vi "Do.vi"(8 "error in (no error)":errorcluster, 10 "Actor in":refnum<class "Actor.lvclass">, 11 "Initiate Sample Transfer Msg":refnum<class "Initiate Sample Transfer Msg.lvclass">) -> (0 "error out":errorcluster, 2 "Actor out":refnum<class "Actor.lvclass">)   [LabVIEW 2015, in "cRIO-Carbondioxide.lvlib" / "cRIO-CO2.lvlib" / "Initiate Sample Transfer Msg.lvclass"]
doc: "This VI delivers the message to the actor by calling the appropriate method(s) on the actor."
uses:
  Initiate Sample Transfer Msg.lvclass
  <vilib>/ActorFramework/Actor/Actor.lvclass
  cRIO-CO2/cRIO-CO2.lvclass
  Initiate Sample Transfer Msg.lvclass/Initiate Sample Transfer Msg.ctl
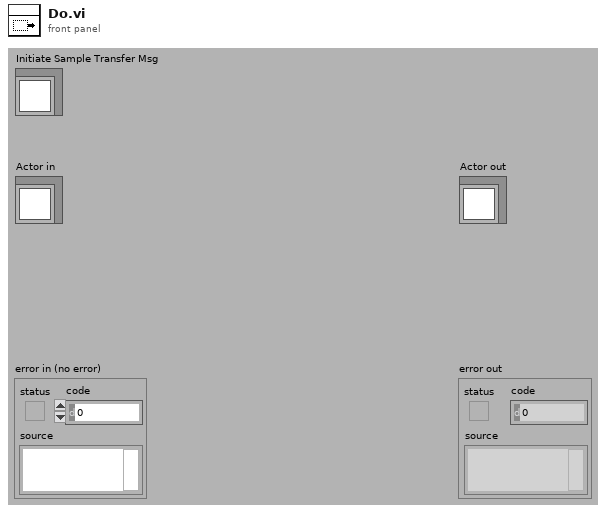
[diagram p1: front panel]
types:
  T1 = typedef "Sample Transfer Container Enumerator.ctl" = enum16{"None", "Sample 1", "Sample 2", "Sample 3", "Sample 4", "Sample 5", "Storage 01", "Storage 02", "Storage 03", "Storage 04", "Storage 05", "Storage 06", "Storage 07", "Storage 08", "Storage 09", "Storage 10", "Storage 11", "Storage 12", "Syringe", "Undefined"}
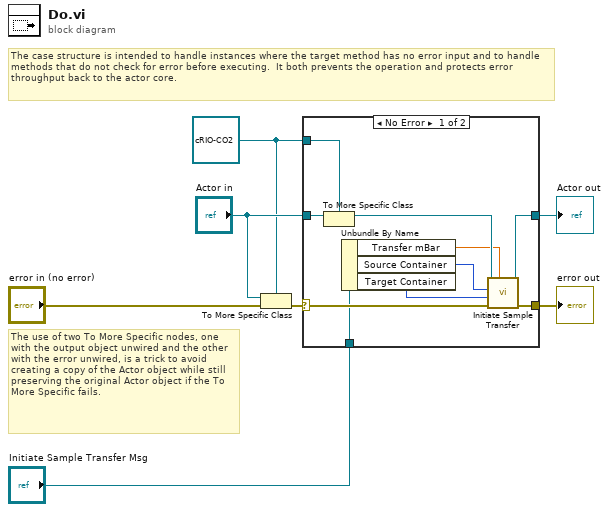
[diagram p0: block diagram]
diagram:
  w2 = refnum<class "cRIO-CO2.lvclass"> refnum ("Actor in")
  # "The use of two To More Specific nodes, one with the output object unwired and the other with the error unwired, is a trick to avoid creating a copy of the Actor object while still preserving the original Actor object if the To More Specific fails."
  # "The case structure is intended to handle instances where the target method has no error input and to handle methods that do not check for error before executing.  It both prevents the operation and protects error throughput back to the actor core."
  n1 = To More Specific Class(target class=w2, reference="Actor in", error in="error in (no error)") -> (error out=w6:errorcluster)  [unwired: 1 out]
  n2 = case shown="No Error" w6 {
    selector: w6 -> [w16 w19]
    tunnel: [w17 w19] -> w5
    tunnel: [w12 w18] -> w4
    tunnel: "Actor in" -> [w15 w18]
    tunnel: w2 -> [w14 _]
    tunnel: "Initiate Sample Transfer Msg" -> [w11 _]
    frame No Error {
      n3 = To More Specific Class(target class=w14, reference=w15) -> (specific class reference=w13:refnum<class "cRIO-CO2.lvclass">)  [unwired: 1 in, 1 out]
      n4 = Unbundle By Name(w11) -> ("Transfer mBar"=w10:dbl, "Source Container"=w8:T1, "Target Container"=w9:T1)
      n5 = call "Initiate Sample Transfer.vi"("Transfer mBar"=w10, "error in (no error)"=w16, "Target Container"=w9, "Source Container"=w8, "cRIO-CO2 in"=w13) -> ("error out"=w17:errorcluster, "cRIO-CO2 out"=w12:refnum<class "cRIO-CO2.lvclass">)  [unwired: 4 in, 1 out]
    }
    frame Error {
      # "If type check fails, pass the original object out again."
    }
  }
  "error out" <- w5
  "Actor out" <- w4
